vi "Get OS Install Date.vi"(8 "error in (no error)":errorcluster) -> (0 "error out":errorcluster, 2 "found?":bool, 3 "OS install date":string)   [LabVIEW 2013]
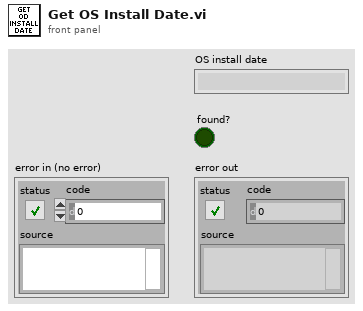
[diagram p1: front panel]
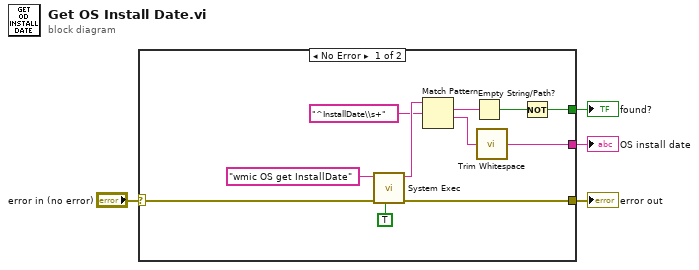
[diagram p0: block diagram]
diagram:
  n1 = case shown="No Error" "error in (no error)" {
    selector: "error in (no error)" -> [w5 w16]
    tunnel: [w10 _] -> w4
    tunnel: [w7 _] -> w3
    tunnel: [w6 w16] -> w2
    frame No Error {
      n2 = call <vilib>:"System Exec.vi"("run minimized? (F)"=TRUE, "error in (no error)"=w5, "command line"="wmic OS get InstallDate") -> ("error out"=w6:errorcluster, "standard output"=w13:string)  [unwired: 5 in, 2 out]
      n3 = Match Pattern(string=w13, regular expression="^InstallDate\\s+") -> (match substring=w9:string, after substring=w11:string)  [unwired: 1 in, 2 out]
      n4 = Empty String/Path?(string/path=w9) -> (empty?=w8:bool)
      n5 = call <vilib>:"Trim Whitespace.vi"("string"=w11) -> ("trimmed string"=w10:string)  [unwired: 1 in]
      n6 = Not(x=w8) -> (.not. x?=w7:bool)
    }
    frame Error {
    }
  }
  "OS install date" <- w4
  "found?" <- w3
  "error out" <- w2
